vi "Get Class Ancestors.vi"(8 "error in (no error)":errorcluster, 11 "Class ID":string) -> (0 "error out":errorcluster, 3 "Class Ancestor IDs[]":string[](array[string]))   [LabVIEW 2023]
doc: "<b> </b> <b> </b>\n© 2017 Q Software Innovations, LLC\nwritten by Quentin \"Q\" Alldredge\nproduced in LabVIEW 2015\n\nsupport@qsoftwareinnovations.com\nwww.qsoftwareinnovations.com\n\nAll rights reserved.\n\nRedistribution and use in source and binary forms, with or without modification, are permitted provided that the following conditions are met:\n\n * Redistributions of source code must retain the above copyright notice, this list of conditions and the following disclaimer.\n * Redistributions in binary form must reproduce the above copyright notice, this list of conditions and the following disclaimer in the documentation and/or other materials provided with the distribution.\n * Neither the name of Q Software Innovations, LLC. nor the names of its contributors may be used to endorse or promote products derived from this software without specific prior written permission.\n\nTHIS SOFTWARE IS PROVIDED BY THE COPYRIGHT HOLDERS AND CONTRIBUTORS \"AS IS\" AND ANY EXPRESS OR IMPLIED WARRANTIES, INCLUDING, BUT NOT LIMITED TO, THE IMPLIED WARRANTIES OF MERCHANTABILITY AND FITNESS FOR A PARTICULAR PURPOSE ARE DISCLAIMED. IN NO EVENT SHALL THE COPYRIGHT OWNER OR CONTRIBUTORS BE LIABLE FOR ANY DIRECT, INDIRECT, INCIDENTAL, SPECIAL, EXEMPLARY, OR CONSEQUENTIAL DAMAGES (INCLUDING, BUT NOT LIMITED TO, PROCUREMENT OF SUBSTITUTE GOODS OR SERVICES; LOSS OF USE, DATA, OR PROFITS; OR BUSINESS INTERRUPTION) HOWEVER CAUSED AND ON ANY THEORY OF LIABILITY, WHETHER IN CONTRACT, STRICT LIABILITY, OR TORT (INCLUDING NEGLIGENCE OR OTHERWISE) ARISING IN ANY WAY OUT OF THE USE OF THIS SOFTWARE, EVEN IF ADVISED OF THE POSSIBILITY OF SUCH DAMAGE."
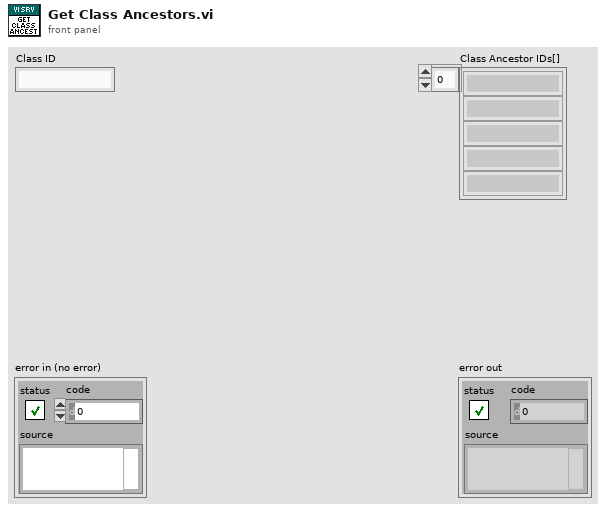
[diagram p1: front panel]
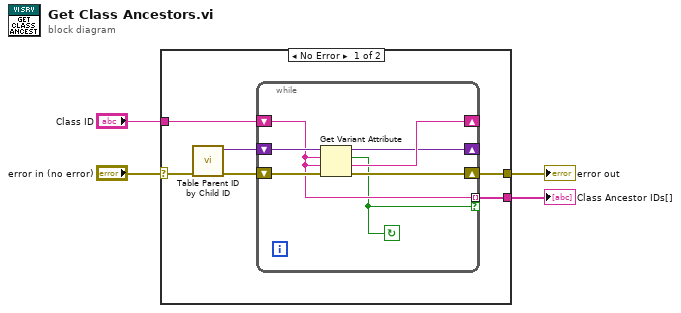
[diagram p0: block diagram]
diagram:
  n1 = case shown="No Error" "error in (no error)" {
    selector: "error in (no error)" -> [w10 w18]
    tunnel: [w6 w18] -> w3
    tunnel: "Class ID" -> [w7 _]
    tunnel: [w5 _] -> w1
    frame No Error {
      n2 = call "Table Parent ID by Child ID.vi"("error in (no error)"=w10) -> ("error out"=w8:errorcluster, "Table Parent ID by Child ID"=w9:variant)  [unwired: 9 in]
      n3 = while {
        shift-right: [w13] -> _
        shift-left: w9 -> [w17]
        shift-right: [w14] -> w6
        shift-left: w8 -> [w16]
        shift-right: [w15] -> _
        shift-left: w7 -> [w12]
        tunnel: [w12] -> w5 mode=indexing if=w11
        stop <- w11 continue-if-true
        n4 = Get Variant Attribute(Variant=w17, name=w12, default value (empty Variant)=w12, error in=w16) -> (duplicate Variant=w13:variant, found=w11:bool, value=w15:string, error out=w14:errorcluster)
      }
    }
    frame Error {
    }
  }
  "error out" <- w3
  "Class Ancestor IDs[]" <- w1
